vi "ForebrainArbiter.vi"(5 "Beh2Input":dbl[](array[numeric]), 7 "HypoInput":dbl[](array[numeric]), 11 "Beh3Input":dbl[](array[numeric])) -> (6 "ForebrainActCom":dbl[](array[numeric]))   [LabVIEW 2010]
doc: "This VI arbitrates command input from theNeo-Cortex, and Hypothallumus THINK processes and conducts a voting poll arbitor with input from each to determine the one output command.\n\nInputs: 90 cell arrays of weighted direction commands \n\nOutput: Cluster of desried velocity and direction"
uses:
  6-OCU Neurons/MainControls.ctl
  6-OCU Neurons/6.1-UDP Saitek.ctl
  6-OCU Neurons/MDF Array LatLong.ctl
  6-OCU Neurons/MDF LatLong.ctl
  4-High Neurons/4.1.0-Datatype Typedef.ctl
  4-High Neurons/4.1.2-Act Neuron TD.ctl
  4-High Neurons/4.1-Act Control Typedef.ctl
  5.0-Global.vi
panel:
  out "5.7.1 Main Controls":T1 {"5.1.1 MDF GPS 2"."Latitude (waypoint)" format="%#_8g"; "5.1.1 MDF GPS 2"."Longitude  (waypoint)" format="%#_8g"; "6.1-Saitek Controller"."Right" scale=-32767.0..32767.0; "6.1-Saitek Controller"."Left" scale=-32767.0..32767.0; "6.1-Saitek Controller"."Yaw" scale=-32767.0..32767.0; "6.1-Saitek Controller"."Roll" scale=-32767.0..32767.0; "6.1-Saitek Controller"."Pitch" scale=-32767.0..32767.0}
  out "Act":bool
  out "Waveform Graph":dbl[][](graph)
  # "This subVI takes the four\nBehavior commands; three from the Neo-Cortex \nand one from theHypoThallumus and\naverages them"
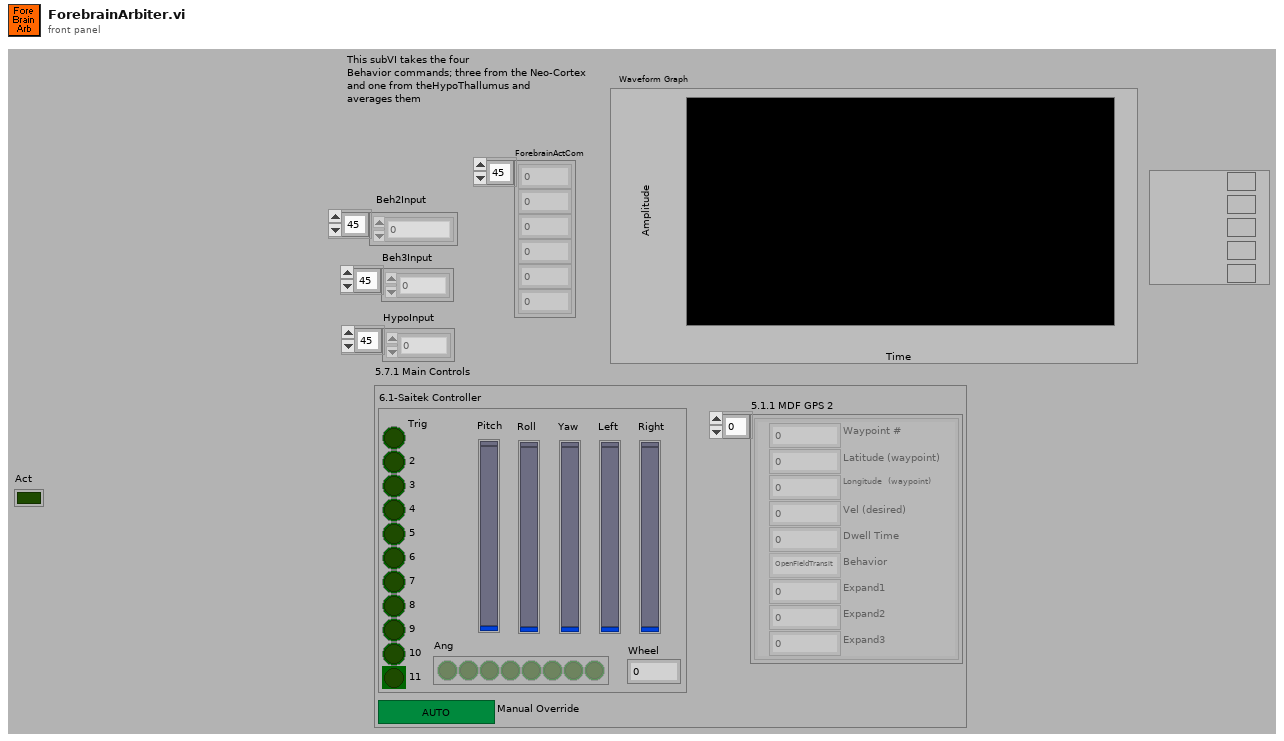
[diagram p1: front panel]
types:
  T1 = typedef "MainControls.ctl" = cluster{"6.1-Saitek Controller":T2, "Manual Override":bool, "5.1.1 MDF GPS 2":T3}
  T2 = typedef "6.1-UDP Saitek.ctl" = cluster{"Trig":bool, "2":bool, "3":bool, "4":bool, "5":bool, "6":bool, "7":bool, "8":bool, "9":bool, "10":bool, "11":bool, "Pitch":i32, "Ang":bool[], "Wheel":dbl, "Roll":i32, "Yaw":i32, "Left":i32, "Right":i32}
  T3 = typedef "MDF Array LatLong.ctl" = T4[]
  T4 = typedef "MDF LatLong.ctl" = cluster{"Waypoint #":dbl, "Latitude (waypoint)":ext, "Longitude  (waypoint)":ext, "Vel (desired)":dbl, "Dwell Time":dbl, "Behavior":enum16{"OpenFieldTransit", "WallFollow", "LaneFollow", "ManualMode"}, "Expand1":dbl, "Expand2":dbl, "Expand3":dbl}
  T5 = typedef "4.1.0-Datatype Typedef.ctl" = enum16{"4.1.0-Empty Data", "4.1.1-Joystick Data", "4.1.2-Behavioral Data"}
  T6 = typedef "4.1.2-Act Neuron TD.ctl" = cluster{"Speed By Path":dbl[]}
  T7 = typedef "4.1-Act Control Typedef.ctl" = cluster{"4.1.0 Data":variant, "Type of Data":T5, "E-Stop":bool, "Restart":bool, "New IP":bool, "Begin":bool, "Time":i32, "Shutdown":bool}
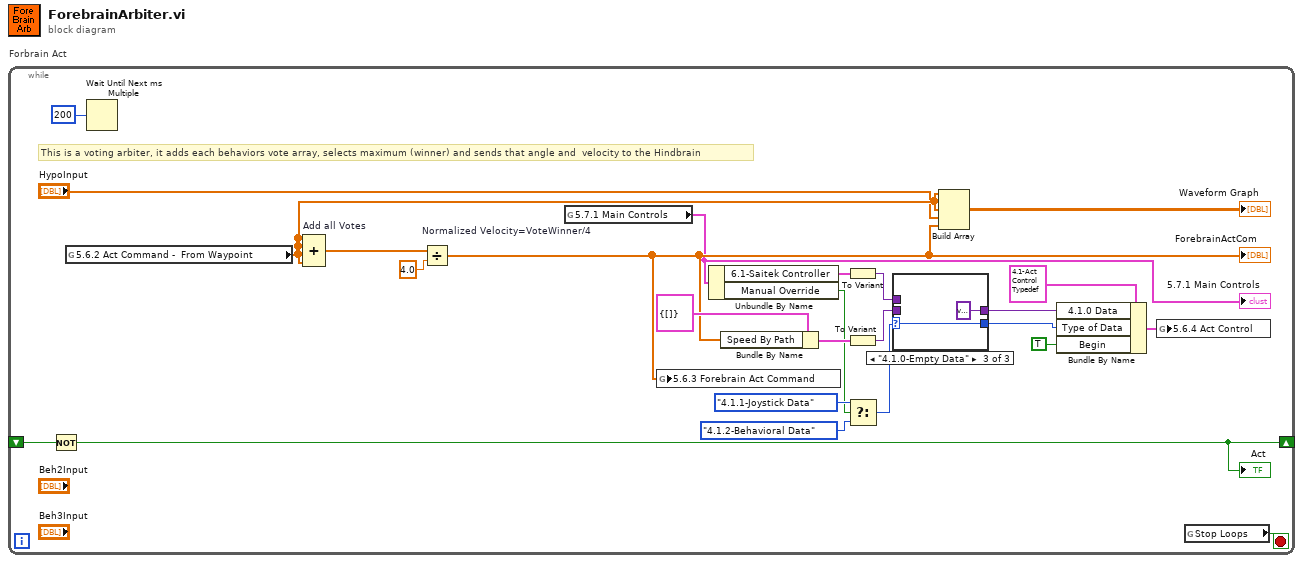
[diagram p0: block diagram]
diagram:
  n1 = while "Forbrain Act" {
    shift-right: [w23] -> _
    shift-left: _ -> [w24]
    stop <- w9 stop-if-true
    # "This is a voting arbiter, it adds each behaviors vote array, selects maximum (winner) and sends that angle and  velocity to the Hindbrain"
    n2 = Not(x=w24) -> (.not. x?=w23:bool)
    "Act" <- w23
    n3 = global read "5.0-Global.vi" "5.6.2 Act Command -  From Waypoint"() -> (w22:dbl[])
    n4 = Wait Until Next ms Multiple(millisecond multiple=u32 200 ("milliseconds to wait")) -> ()  [unwired: 1 out]
    n5 = Compound Arithmetic op=ADD "Add all Votes"(w22, w22, w22, w22) -> (w19:dbl[])
    n6 = Divide "Normalized Velocity=VoteWinner/4"(x=w19, y=4.0) -> (x/y=w16:dbl[])
    "ForebrainActCom" <- w16
    n7 = global read "5.0-Global.vi" "5.7.1 Main Controls"() -> (w11:T1)
    "5.7.1 Main Controls" <- w11
    n8 = global write "5.0-Global.vi" "5.6.3 Forebrain Act Command"(w16) -> ()
    n9 = Unbundle By Name(w11) -> ("6.1-Saitek Controller"=w10:T2, "Manual Override"=w6:bool)
    n10 = Bundle By Name(cluster=T6 {"Speed By Path"=[]} ("Forebrain Act Neurons"), "Speed By Path"=w16) -> (w15:T6)
    n11 = To Variant(anything=w10) -> (Variant=w5:variant)
    n12 = To Variant(anything=w15) -> (Variant=w3:variant)
    n13 = Select(t=4.1.0-Datatype_Typedef."4.1.1-Joystick Data" ("Type of Data"), s=w6, f=4.1.0-Datatype_Typedef."4.1.2-Behavioral Data" ("Type of Data")) -> (s? t:f=w2:T5)
    n14 = case shown="\"4.1.0-Empty Data\"" w2 {
      selector: w2 -> [w26 w28 w30]
      tunnel: w5 -> [w27 _ _]
      tunnel: [w27 w29 variant ("Variant")] -> w4
      tunnel: w3 -> [_ w29 _]
      tunnel: [w26 w28 w30] -> w1
      frame "4.1.1-Joystick Data" {
      }
      frame "4.1.2-Behavioral Data" {
      }
      frame "4.1.0-Empty Data" {
      }
    }
    n15 = Build Array "Build Array"(w22, w22, w22, "HypoInput", w16) -> (→"Waveform Graph":dbl[][])
    n16 = Bundle By Name(cluster=T7 {"4.1.0 Data"=variant, "Type of Data"=enum."4.1.0-Empty Data", "E-Stop"=FALSE, "Restart"=FALSE, "New IP"=FALSE, "Begin"=FALSE, "Time"=0, "Shutdown"=FALSE} ("5.6.4 Act Control"), "4.1.0 Data"=w4, "Type of Data"=w1, "Begin"=TRUE) -> (w13:T7)
    n17 = global write "5.0-Global.vi" "5.6.4 Act Control"(w13) -> ()
    n18 = global read "5.0-Global.vi" "Stop Loops"() -> (w9:bool)
  }
